vi "sr-flip-flop-nand.vi"(8 "Reset":bool, 11 "Set":bool) -> (0 "!Q":bool, 3 "Q":bool)   [LabVIEW 2024]
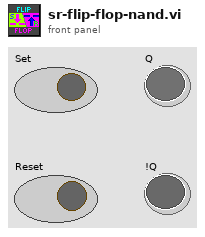
[diagram p1: front panel]
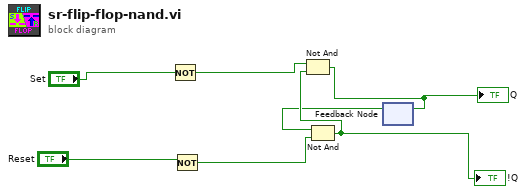
[diagram p0: block diagram]
diagram:
  n1 = Not(x="Set") -> (.not. x?=w3:bool)
  n2 = Not(x="Reset") -> (.not. x?=w1:bool)
  n3 = feedback #1() -> (w6:bool)  [unwired: 1 in]
  n4 = Not And(1:w1, 2:w6) -> (0:w7:bool)
  "!Q" <- w7
  n5 = Not And(1:w7, 2:w3) -> (0:w5:bool)
  "Q" <- w5
  n6 = feedback-in #1(w5) -> ()
